vi "Get Cursor data (SubVI).vi"(8 "Signal":dbl[](array[numeric]), 9 "Time":dbl[](array[numeric]), 10 "Time position":dbl[](array[numeric]), 11 "XYGraph Refnum":refnum<vi>) -> (0 "Signal cursor":dbl[](array[numeric]), 1 "Time cursor":dbl[](array[numeric]), 2 "Index cursor":dbl[](array[numeric]), 5 "?":cluster{"all rows":dbl[], "all rows":dbl[]}(graph))   [LabVIEW 2014]
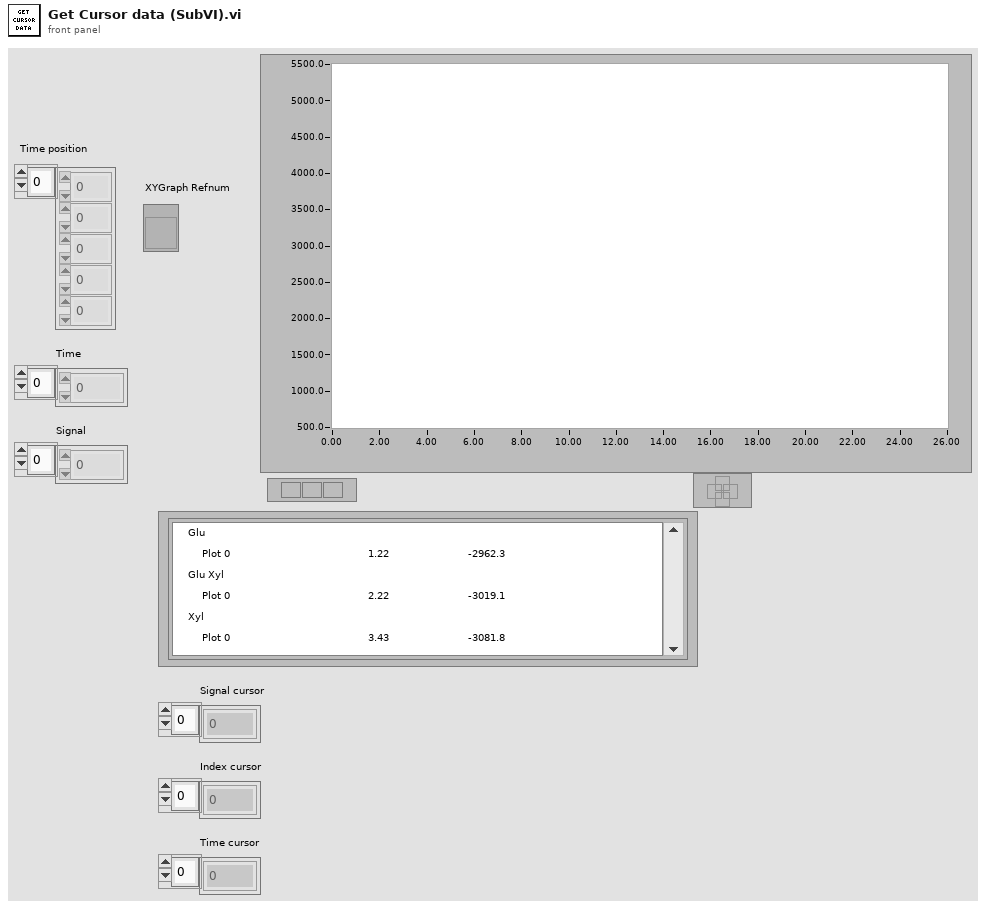
[diagram p1: front panel]
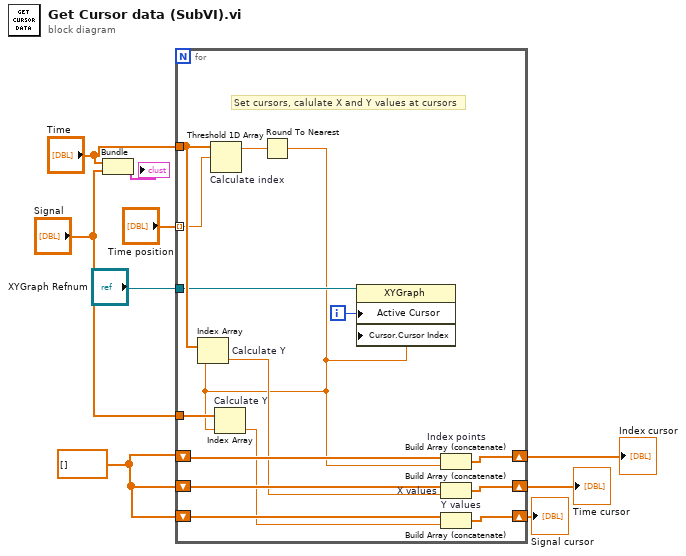
[diagram p0: block diagram]
diagram:
  w2 = dbl[] []
  n1 = Bundle("Time"="Time", "Signal"="Signal") -> (→"?":cluster{"Time":dbl[], "Signal":dbl[]})  [unwired: 1 in]
  n2 = for {
    tunnel: "Time" -> [w16]
    tunnel: "Signal" -> [w17]
    shift-right: [w23] -> w7
    shift-left: w2 -> [w22]
    shift-right: [w21] -> w5
    shift-left: w2 -> [w20]
    shift-right: [w19] -> w6
    shift-left: w2 -> [w18]
    tunnel: "XYGraph Refnum" -> [w13]
    tunnel: "Time position" -> [w12] mode=indexing
    i -> [w11]
    # "Set cursors, calulate X and Y values at cursors"
    n3 = Threshold 1D Array "Calculate index"(2:w12, 3:w16) -> (0:w24:dbl)  [unwired: 1 in]
    n4 = Round To Nearest(number=w24) -> (nearest integer value=w10:dbl)
    n5 = Index Array "Calculate Y"(array=w16, index=w10) -> (element=w15:dbl)
    n6 = Index Array "Calculate Y"(array=w17, index=w10) -> (element=w14:dbl)
    n7 = property on="Property Node" class="XYGraph"(reference=w13, "Active Cursor"=w11, "Cursor.Cursor Index"=w10) -> ()  [unwired: 1 in, 2 out]
    n8 = Build Array (concatenate) "Index points"(w22, w10) -> (w23:dbl[])
    n9 = Build Array (concatenate) "X values"(w20, w15) -> (w21:dbl[])
    n10 = Build Array (concatenate) "Y values"(w18, w14) -> (w19:dbl[])
  }
  "Index cursor" <- w7
  "Signal cursor" <- w6
  "Time cursor" <- w5
